vi "lab.vi"(0 "String input":string) -> ()   [LabVIEW 2013]
panel:
  out "Slope distance":dbl
  out "V":dbl
  out "Hz":dbl
  out "Slope distance":string
  out "V":string
  out "Hz":string
  out "before substring":string
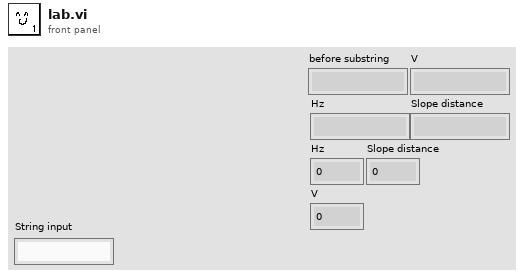
[diagram p1: front panel]
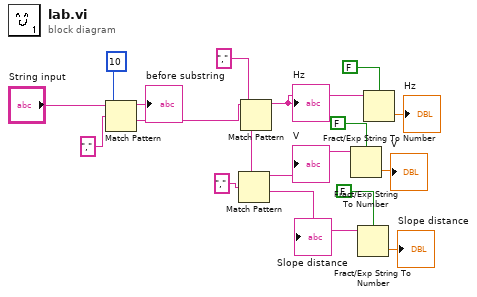
[diagram p0: block diagram]
diagram:
  n1 = Match Pattern(string="String input", regular expression=",", offset (0)=10) -> (before substring=→"before substring":string, after substring=w13:string)  [unwired: 2 out]
  n2 = Match Pattern(string=w13, regular expression=",") -> (before substring=w9:string, after substring=w11:string)  [unwired: 1 in, 2 out]
  "Hz" <- w9
  n3 = Match Pattern(string=w11, regular expression=",") -> (before substring=w8:string, after substring=w7:string)  [unwired: 1 in, 2 out]
  "V" <- w8
  "Slope distance" <- w7
  n4 = Fract/Exp String To Number(use system decimal point (T)=FALSE, string=w8) -> (number=→"V":dbl)  [unwired: 2 in, 1 out]
  n5 = Fract/Exp String To Number(use system decimal point (T)=FALSE, string=w7) -> (number=→"Slope distance":dbl)  [unwired: 2 in, 1 out]
  n6 = Fract/Exp String To Number(use system decimal point (T)=FALSE, string=w9) -> (number=→"Hz":dbl)  [unwired: 2 in, 1 out]
